vi "Filter Target Names.vi"(7 "Target Name":string="My Computer", 8 "error in (no error)":errorcluster, 11 "Project Sync Tools in":refnum<class "Project Sync Tools.lvclass">) -> (0 "error out":errorcluster, 2 "Filtered Names":string[](array[string]), 3 "Project Sync Tools out":refnum<class "Project Sync Tools.lvclass">)   [LabVIEW 2019, in "Project Sync Tools.lvclass"]
uses:
  Project Sync Tools.lvclass
  <userlib>/_OpenG.lib/array/array.llb/Filter 1D Array with Scalar (String)__ogtk.vi
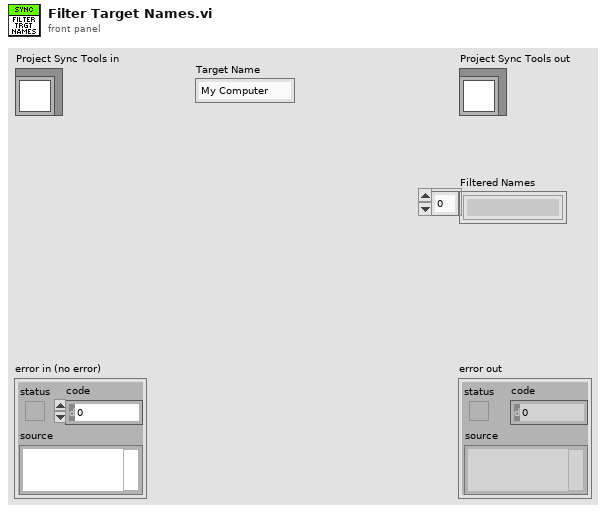
[diagram p1: front panel]
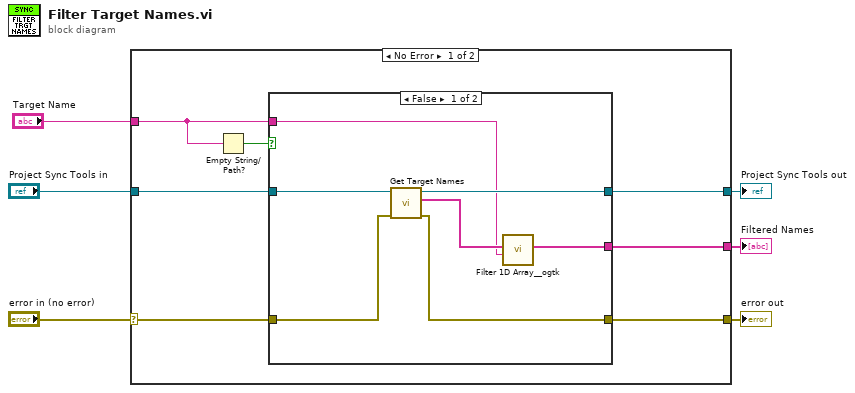
[diagram p0: block diagram]
diagram:
  n1 = case shown="No Error" "error in (no error)" {
    selector: "error in (no error)" -> [w10 w24]
    tunnel: [w9 w24] -> w5
    tunnel: [w12 w23] -> w3
    tunnel: "Project Sync Tools in" -> [w13 w23]
    tunnel: "Target Name" -> [w8 _]
    tunnel: [w11 _] -> w1
    frame No Error {
      n2 = Empty String/Path?(string/path=w8) -> (empty?=w7:bool)
      n3 = case shown="False" w7 {
        tunnel: w13 -> [w19 w22]
        tunnel: [w18 w22] -> w12
        tunnel: [w17 _] -> w11
        tunnel: w10 -> [w16 w21]
        tunnel: [w15 w21] -> w9
        tunnel: w8 -> [w14 _]
        frame False {
          n4 = call "Get Target Names.vi"("error in (no error)"=w16, "Project Sync Tools in"=w19) -> ("error out"=w15:errorcluster, "Targets names"=w20:string[], "Project Sync Tools out"=w18:refnum<class "Project Sync Tools.lvclass">)  [unwired: 7 in]
          n5 = call-poly <userlib>:"Filter 1D Array__ogtk.vi"("items to filter"=w14, "array"=w20) -> ("filtered array"=w17:string[])  [unwired: 4 in, 1 out]
        }
        frame True {
        }
      }
    }
    frame Error {
    }
  }
  "error out" <- w5
  "Project Sync Tools out" <- w3
  "Filtered Names" <- w1
